vi "uTransport_SendMsg Core.vi"(8 "error in (no error)":errorcluster, 10 "Msg":refnum<class "uMsg.lvclass">, 11 "uClient_Publisher in":refnum<class "uClient_Publisher.lvclass">) -> (0 "error out":errorcluster, 3 "uClient_Publisher out":refnum<class "uClient_Publisher.lvclass">)   [LabVIEW 2023, in "uLib.lvlib" / "uClient_Publisher.lvclass"]
uses:
  uClient_Publisher.lvclass
  uMsg/uMsg/uMsg.lvclass
  uClient_Publisher.lvclass/uClient_Publisher.ctl
  uMsg/uMsg/uMsg.lvclass/uMsg.ctl
  uData/uData/uData.lvclass/uData.ctl
  uData/uData/Set Tag.vi
  uMsg/uMsg/uMsg Update Timestamp.vi
  uMsg/uMsg/uMsg Rename CMD.vi
  uMsg/uMsg/uMsg Get CMD.vi
  uMsg/uMsg/Write Payload.vi
  uMsg/uMsg/uMsg Create.vi
  uData/uData/Condition Tag Name.vi
  uData/uData/Blank Key Reserved String.vi
  uData/uData/uData.lvclass
  uTransport/uTransport/uTransport.lvclass
  uStringManipulation/uStringManipulation/uStringManipulation.lvclass
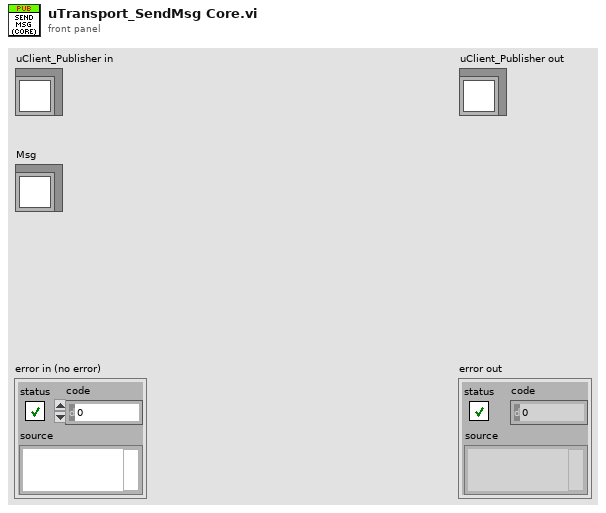
[diagram p1: front panel]
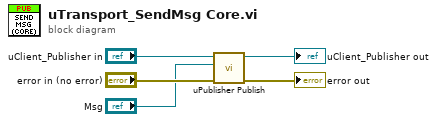
[diagram p0: block diagram]
diagram:
  n1 = call "uPublisher Publish.vi"("error in (no error)"="error in (no error)", "uMsg"="Msg", "uClient_Publisher in"="uClient_Publisher in") -> ("error out"=→"error out":errorcluster, "uClient_Publisher out"=→"uClient_Publisher out":refnum<class "uClient_Publisher.lvclass">)  [unwired: 7 in]
